vi "Readable String.vi"(11 "Time Condition in":refnum<class "Time Condition.lvclass">) -> (2 "String":string)   [LabVIEW 2020, in "VolatusSeq.lvlib" / "Time Condition.lvclass"]
uses:
  Time Condition.lvclass
  Time Condition.lvclass/Time Condition.ctl
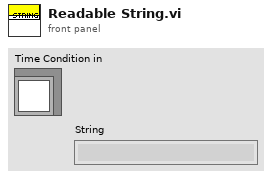
[diagram p1: front panel]
types:
  T1 = typedef "VolatusSeqConfig.lvlib/Timer.ctl" = enum16{"Sequence", "State", "Wall"}
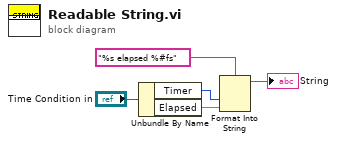
[diagram p0: block diagram]
diagram:
  n1 = Unbundle By Name("Time Condition in") -> ("Timer"=w3:T1, "Elapsed"=w2:dbl)
  n2 = Format Into String(format string="%s elapsed %#fs", w3, w2) -> (resulting string=→"String":string)  [unwired: 2 in, 1 out]
